vi "Keith 7001 Channel String.vi"(1 "channel list":T1(array[cluster])) -> (0 "?":string)   [LabVIEW 2019]
doc: "This VI converts an array of channels and memory locations into a string to be used by other VIs requiring a channel list or a scan list such as \"open/close channels\"."
panel:
  # "memory location\nstandard channel"
  # "matrix card\nnon-matrix card"
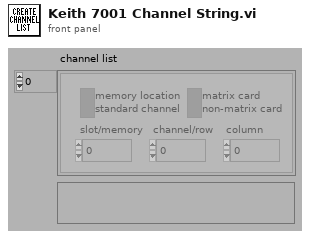
[diagram p1: front panel]
types:
  T1 = cluster{"slot/memory":i16, "channel/row":i16, "column":i16, bool, bool}[]
  T2 = cluster{"slot/memory":i16, "channel/row":i16, "column":i16, bool, bool}
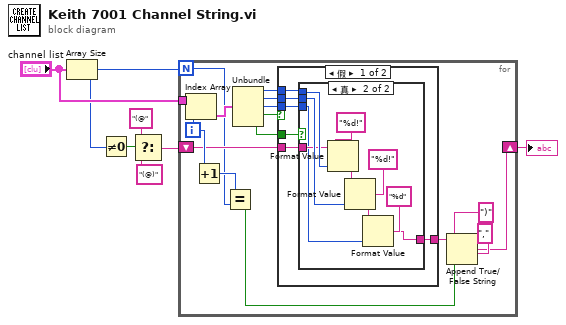
[diagram p0: block diagram]
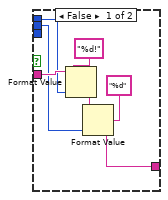
[diagram p2: hidden frame]
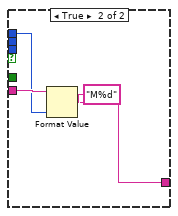
[diagram p3: hidden frame]
diagram:
  n1 = Array Size(array="channel list") -> (size(s)=w2:i32)
  n2 = Not Equal To 0?(x=w2) -> (x != 0?=w4:bool)
  n3 = Select(t="(@", s=w4, f="(@)") -> (s? t:f=w3:string)
  n4 = for {
    N: w2 -> [w8]
    tunnel: "channel list" -> [w23]
    shift-right: [w9] -> w1
    shift-left: w3 -> [w19]
    i -> [w22]
    n5 = Index Array(array=w23, index=w22) -> (element=w21:T2)
    n6 = Increment(x=w22) -> (x+1=w14:i32)
    n7 = Equal?(x=w14, y=w8) -> (x = y?=w12:bool)
    n8 = Unbundle(w21) -> ("slot/memory"=w18:i16, "channel/row"=w16:i16, "column"=w15:i16, w20:bool, w17:bool)
    n9 = case shown="假" w20 {
      tunnel: w19 -> [w28 w49]
      tunnel: w18 -> [w27 w48]
      tunnel: [w24 w47] -> w13
      tunnel: w17 -> [w29 _]
      tunnel: w16 -> [w26 _]
      tunnel: w15 -> [w25 _]
      frame False {
        n10 = case shown="真" w29 {
          tunnel: w28 -> [w36 w41]
          tunnel: w27 -> [w32 w43]
          tunnel: w26 -> [w31 w42]
          tunnel: [w30 w38] -> w24
          tunnel: w25 -> [_ w37]
          frame False {
            n11 = Format Value(string ("")=w36, format string="%d!", value (0)=w32) -> (output string=w34:string)
            n12 = Format Value(string ("")=w34, format string="%d", value (0)=w31) -> (output string=w30:string)
          }
          frame True {
            n13 = Format Value(string ("")=w41, format string="%d!", value (0)=w43) -> (output string=w45:string)
            n14 = Format Value(string ("")=w45, format string="%d!", value (0)=w42) -> (output string=w39:string)
            n15 = Format Value(string ("")=w39, format string="%d", value (0)=w37) -> (output string=w38:string)
          }
        }
      }
      frame True {
        n16 = Format Value(string ("")=w49, format string="M%d", value (0)=w48) -> (output string=w47:string)
      }
    }
    n17 = Append True/False String(1:w12, 2:",", 3:")", 4:w13) -> (0:w9:string)
  }
  "?" <- w1
